vi "Add Packages to Feed.vi"(0 "Feed Path":path, 5 "Packages Path":path, 11 "error in (no error)":errorcluster) -> (15 "error out":errorcluster)   [LabVIEW 2021, in "Packager Helpers.lvlib"]
uses:
  Packager Helpers.lvlib
  Path Functions/Path Functions.lvlib
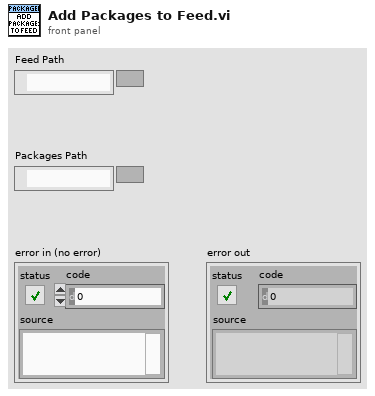
[diagram p1: front panel]
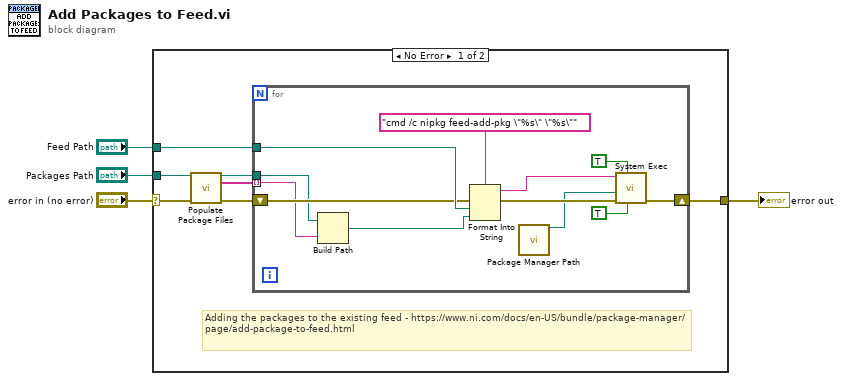
[diagram p0: block diagram]
diagram:
  n1 = case shown="No Error" "error in (no error)" {
    selector: "error in (no error)" -> [w7 w24]
    tunnel: [w11 w24] -> w3
    tunnel: "Feed Path" -> [w10 _]
    tunnel: "Packages Path" -> [w9 _]
    frame No Error {
      # "Adding the packages to the existing feed - https://www.ni.com/docs/en-US/bundle/package-manager/page/add-package-to-feed.html"
      n2 = call "Populate Package Files.vi"("Packages Path"=w9, "error in (no error)"=w7) -> ("Path Out"=w5:path, "Filenames"=w6:string[], "error out"=w8:errorcluster)  [unwired: 11 in]
      n3 = for {
        tunnel: w10 -> [w16]
        shift-right: [w18] -> w11
        shift-left: w8 -> [w15]
        tunnel: w6 -> [w13] mode=indexing
        tunnel: w5 -> [w14]
        n4 = Build Path(base path=w14, name or relative path=w13) -> (appended path=w12:path)
        n5 = Format Into String(format string="cmd /c nipkg feed-add-pkg \"%s\" \"%s\"", error in=w15, w16, w12) -> (resulting string=w21:string, error out=w20:errorcluster)  [unwired: 1 in]
        n6 = call "Package Manager Path.vi"() -> ("Package Manager Path"=w17:path)  [unwired: 15 in]
        n7 = call <vilib>:"System Exec.vi"("run minimized? (F)"=TRUE, "wait until completion? (T)"=TRUE, "error in (no error)"=w20, "working directory"=w17, "command line"=w21) -> ("error out"=w18:errorcluster)  [unwired: 3 in, 3 out]
      }
    }
    frame Error {
    }
  }
  "error out" <- w3
